vi "Aiming with Turning.vi"() -> ()   [LabVIEW 2015]
uses:
  GitHub/2016-Practice-Bot-Code/navX Library v2/navX Library v2.lvlib
panel:
  in  "Button Pressed?":bool
  in  "Case":dbl
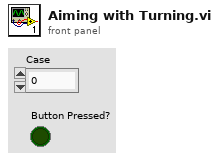
[diagram p1: front panel]
types:
  T1 = typedef "navX Library v2.lvlib/Z900_navX_DeviceTypeDef.ctl" = cluster{"Interface":cluster{"Protocol":T2, "Update Rate (4Hz-60Hz)":u8, "navX Open TypeDef":variant}, "Notify Packet":refnum<notifier>, "Loop VI Refnum":refnum<vi>, "Ready to Close Occurrence Refnum":refnum<k4>}
  T2 = typedef "navX Library v2.lvlib/Z900_navX_ProtocolTypeDef.ctl" = enum16{"SERIAL", "I2C", "SPI"}
  T3 = cluster{"Accel X":dbl, "Accel Y":dbl, "Accel Z":dbl, "Gyro X":dbl, "Gyro Y":dbl, "Gyro Z":dbl, "Mag X":dbl, "Mag Y":dbl, "Mag Z":dbl}
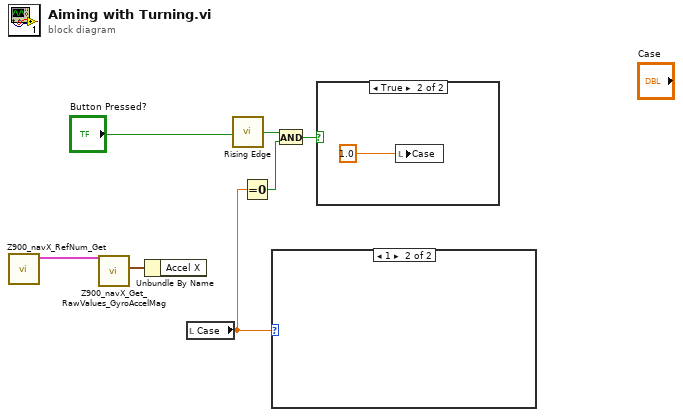
[diagram p0: block diagram]
diagram:
  n1 = call "Z900_navX_RefNum_Get.vi"() -> ("navX Device"=w1:T1)  [unwired: 10 in, 1 out]
  n2 = call "Z900_navX_Get_RawValues_GyroAccelMag.vi"("navX Device"=w1) -> ("Raw Values"=w2:T3)  [unwired: 7 in, 3 out]
  n3 = Unbundle By Name(w2) -> ()  [unwired: 1 out]
  n4 = local read "Case"() -> (w3:dbl)
  n5 = call "Rising Edge.vi"("Button Pressed?"="Button Pressed?") -> ("Bool Output"=w6:bool)
  n6 = Equal To 0?(x=w3) -> (x = 0?=w4:bool)
  n7 = case shown="1" w3 {
    frame 0, Default {
      # "DO NOTHING"
    }
    frame 1 {
    }
  }
  n8 = And(x=w6, y=w4) -> (x .and. y?=w5:bool)
  n9 = case shown="True" w5 {
    frame False {
    }
    frame True {
      n10 = local write "Case"(1.0) -> ()
    }
  }
